vi "SR List FGV.vi"(7 "Operation":T3, 8 "Error In":errorcluster, 9 "Input":variant) -> (0 "Error Out":errorcluster, 2 "list out":T1[](array[typedef]) {"Creation Date" format="%<%x>T"; "Last Updated" format="%<%x>T"})   [LabVIEW 2018]
doc: "Functional global variable that stores and modifies the SR list"
uses:
  Type Defs/FGV States.ctl
  Type Defs/SR Cluster.ctl
  Type Defs/SR Status.ctl
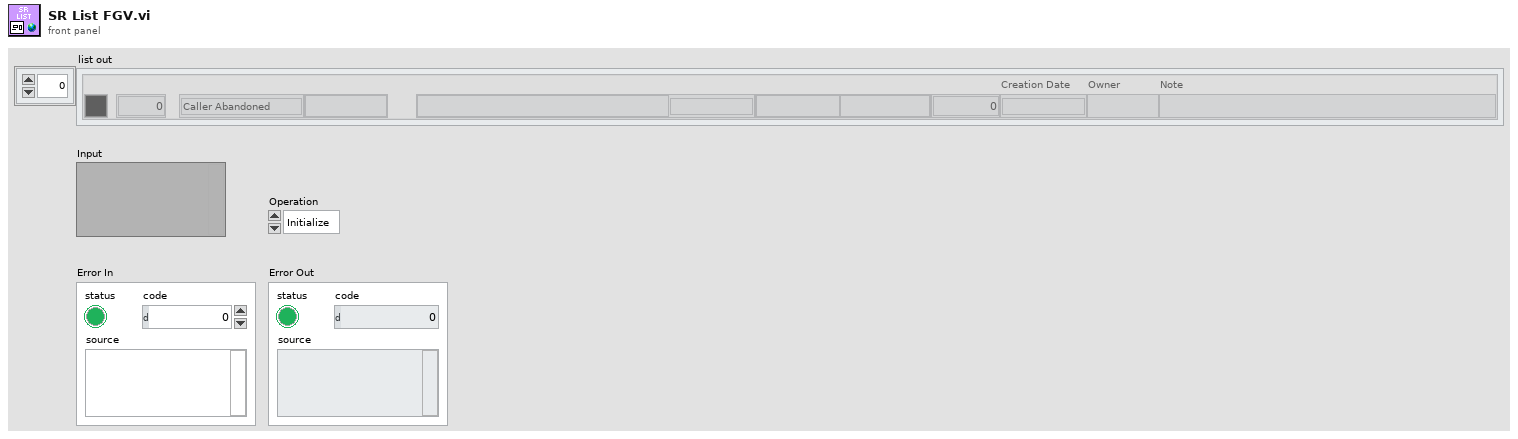
[diagram p1: front panel]
types:
  T1 = typedef "SR Cluster.ctl" = cluster{"Color":u32, "SR Number":i32, "SR Status":T2, "Name":string, "Summary":string, "Last Updated":timestamp, "SR Type":string, "Service Level":string, "Days Open":dbl, "Creation Date":timestamp, "Owner":string, "Note":string}
  T2 = typedef "SR Status.ctl" = enum16{"Caller Abandoned", "Created in Error", "Expired", "Forum Resolved AE", "Forum Resolved Customer", "IN WORK", "IN WORK Collab with AES", "IN WORK Collab with PSE", "IN WORK Collab with SE", "IN WORK Customer Added Note", "IN WORK Escalation", "IN WORK Wait on Customer", "Open", "Potentially Resolved", "Presumed Resolved", "RMA Approved for Return", "RMA Closed", "RMA Closed - DOA", "RMA In Progress", "RMA Open", "RMA Waiting on Customer", "Resolved", "Passed Off"}
  T3 = typedef "FGV States.ctl" = enum16{"Initialize", "Merge", "Write", "Remove", "Read", "Clear"}
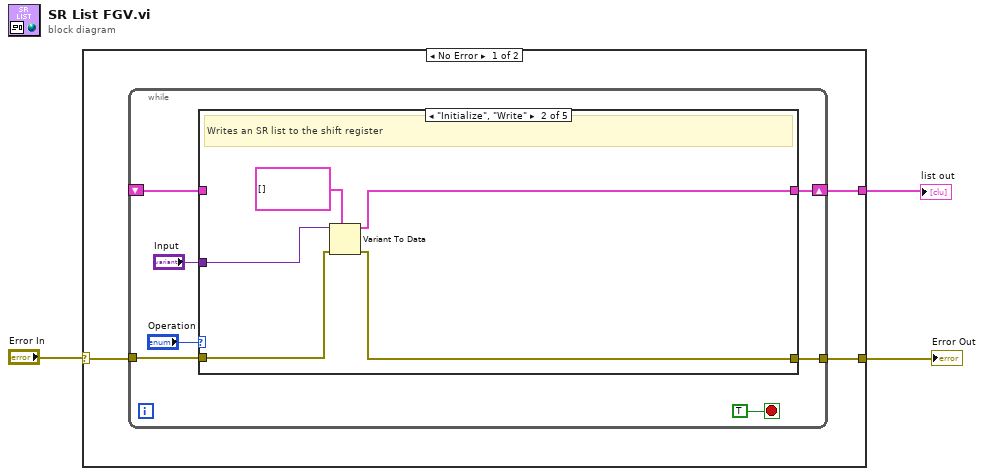
[diagram p0: block diagram]
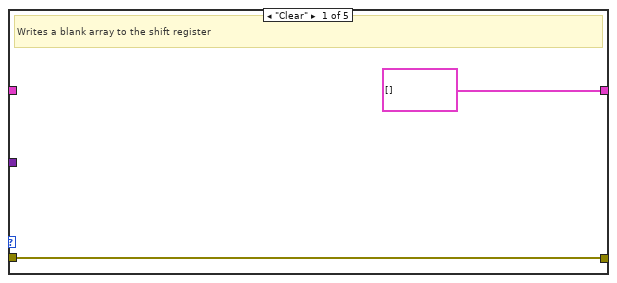
[diagram p2: hidden frame]
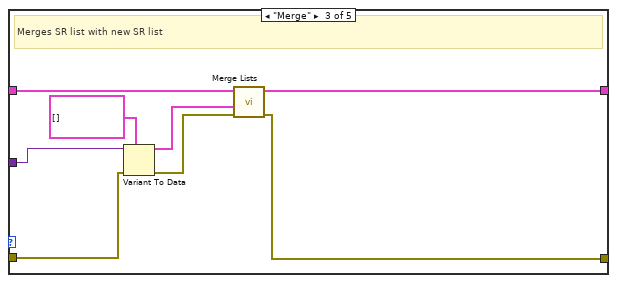
[diagram p3: hidden frame]
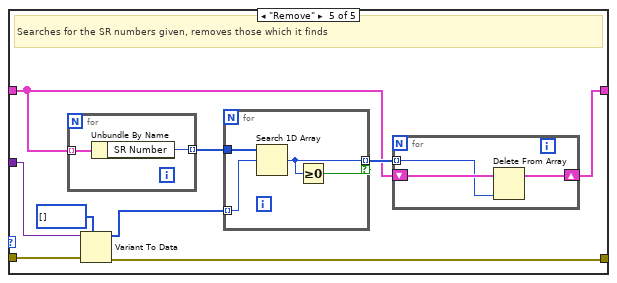
[diagram p5: hidden frame]
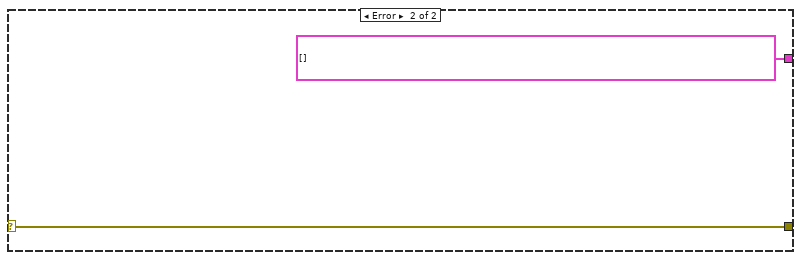
[diagram p6: hidden frame]
diagram:
  n1 = case shown="No Error" "Error In" {
    selector: "Error In" -> [w5 w50]
    tunnel: [w6 T1[] [] ("list out")] -> w3
    tunnel: [w4 w50] -> w1
    frame No Error {
      n2 = while {
        shift-right: [w13] -> w6
        shift-left: _ -> [w12]
        tunnel: w5 -> [w8]
        tunnel: [w7] -> w4
        stop <- TRUE stop-if-true
        n3 = case shown="\"Initialize\", \"Write\"" "Operation" {
          tunnel: [T1[] [] ("List In") w18 w27 w30 w31] -> w13
          tunnel: w12 -> [_ _ w28 w30 w32]
          tunnel: "Input" -> [_ w20 w25 _ w34]
          tunnel: w8 -> [w14 w17 w23 w29 w37]
          tunnel: [w14 w16 w21 w29 w36] -> w7
          frame "Clear" {
            # "Writes a blank array to the shift register"
          }
          frame "Initialize", "Write" {
            # "Writes an SR list to the shift register"
            n4 = Variant To Data(error in=w17, type=T1[] [] ("list in"), Variant=w20) -> (data=w18:T1[], error out=w16:errorcluster)
          }
          frame "Merge" {
            # "Merges SR list with new SR list"
            n5 = Variant To Data(error in=w23, type=T1[] [] ("list in"), Variant=w25) -> (data=w24:T1[], error out=w22:errorcluster)
            n6 = call "Merge Lists.vi"("error in"=w22, "new list in"=w24, "list in"=w28) -> ("error out"=w21:errorcluster, "list out"=w27:T1[])  [unwired: 7 in]
          }
          frame "Read" {
            # "Returns the value currently stored in the shift register"
          }
          frame "Remove" {
            # "Searches for the SR numbers given, removes those which it finds"
            n7 = for {
              tunnel: w32 -> [w41] mode=indexing
              tunnel: [w40] -> w38 mode=indexing
              n8 = Unbundle By Name(w41) -> ("SR Number"=w40:i32)
            }
            n9 = Variant To Data(error in=w37, type=i32[] [], Variant=w34) -> (data=w33:i32[], error out=w36:errorcluster)
            n10 = for {
              tunnel: w33 -> [w42] mode=indexing
              tunnel: w38 -> [w45]
              tunnel: [w44] -> w39 mode=indexing if=w43
              n11 = Search 1D Array(1D array=w45, element=w42) -> (index of element=w44:i32)  [unwired: 1 in]
              n12 = Greater Or Equal To 0?(x=w44) -> (x >= 0?=w43:bool)
            }
            n13 = for {
              tunnel: w39 -> [w47] mode=indexing
              shift-right: [w46] -> w31
              shift-left: w32 -> [w48]
              n14 = Delete From Array(array=w48, index=w47) -> (array with subset deleted=w46:T1[])  [unwired: 1 in, 1 out]
            }
          }
        }
      }
    }
    frame Error {
    }
  }
  "Error Out" <- w1
  "list out" <- w3
